vi "testConnectDisconnect.vi"(8 "error in (no error)":errorcluster) -> (0 "error out":errorcluster)   [LabVIEW 2018]
doc: "This VI test the connection and disconnection of TcpServerCmd and TcpServerTel."
uses:
  <vilib>/addons/_JKI Toolkits/Caraya/classes/Assert/Assert Equal Value_Variant.vi
  src/TcpServer/TcpServer.lvclass
  <vilib>/addons/_JKI Toolkits/Caraya/classes/Test/Test.lvclass
  <vilib>/addons/_JKI Toolkits/Caraya/classes/Assert/Assert.lvclass
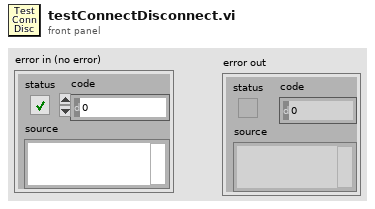
[diagram p1: front panel]
types:
  T1 = cluster{"CmdRead":refnum<user-event>, "EvtRead":refnum<user-event>, "GenRead":refnum<user-event>}
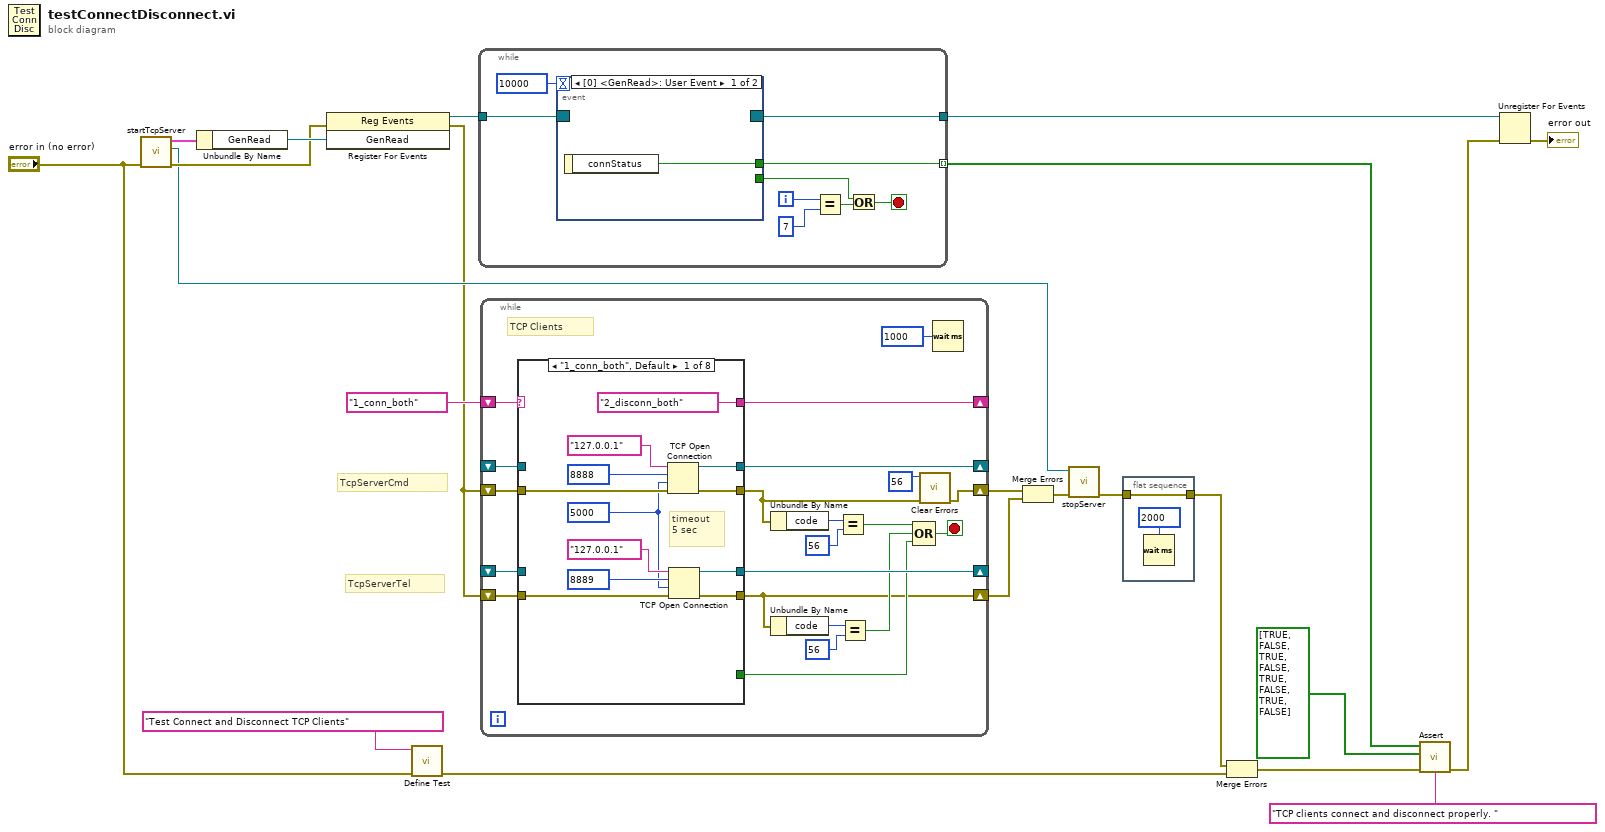
[diagram p0: block diagram]
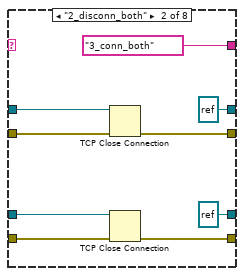
[diagram p2: hidden frame]
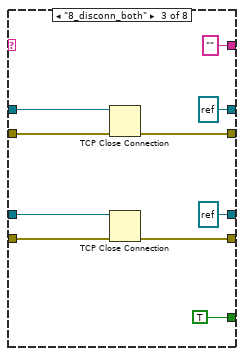
[diagram p3: hidden frame]
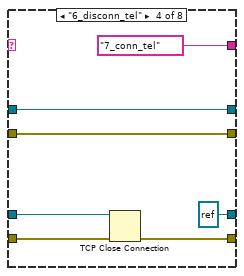
[diagram p4: hidden frame]
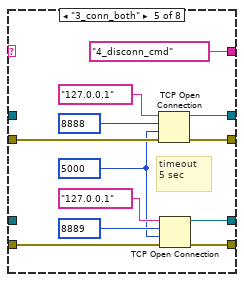
[diagram p5: hidden frame]
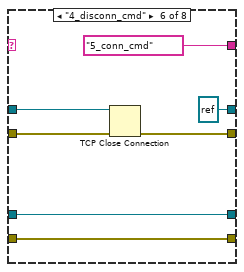
[diagram p6: hidden frame]
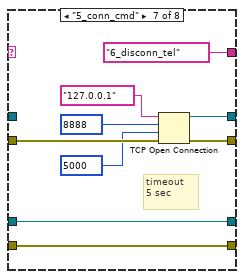
[diagram p7: hidden frame]
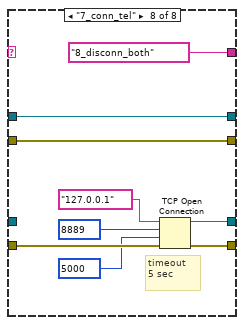
[diagram p8: hidden frame]
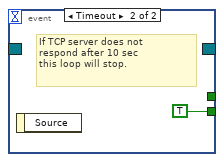
[diagram p9: hidden frame]
diagram:
  # "TcpServerTel"
  # "TcpServerCmd"
  n1 = call "startTcpServer.vi"("error in (no error)"="error in (no error)") -> ("error out"=w14:errorcluster, "TcpServer out"=w10:refnum<class "TcpServer.lvclass">, "UserEvents"=w17:T1)  [unwired: 8 in]
  n2 = Unbundle By Name(w17) -> ("GenRead"=w16:refnum<user-event>)
  n3 = register-events(error in=w14, w16) -> (reference out=w22:refnum<event-registration>, error out=w2:errorcluster)  [unwired: 1 in]
  n4 = call <vilib>:"Define Test.vi"("error in (no error)"="error in (no error)", "Label (VI Title)"="Test Connect and Disconnect TCP Clients") -> ("error out"=w7:errorcluster)  [unwired: 9 in]
  n5 = while {
    tunnel: w22 -> [w31]
    tunnel: [w30] -> w21
    tunnel: [w27] -> w9 mode=indexing
    i -> [w28]
    stop <- w23 stop-if-true
    n6 = event shown="[0] <GenRead>: User Event" {
      selector: w31 -> [_ _]
      dyn-events: [_ _] -> w30
      timeout: 10000 -> [_ _]
      tunnel: [w32 _] -> w27
      tunnel: [_ TRUE] -> w24
      event User Event {
        n7 = event-data() -> ("connStatus"=w32:bool)  [unwired: 1 in]
      }
      event Timeout {
        # "If TCP server does not\nrespond after 10 sec\nthis loop will stop."
        n8 = event-data() -> ()  [unwired: 1 in, 1 out]
      }
    }
    n9 = Equal?(x=w28, y=7) -> (x = y?=w25:bool)
    n10 = Or(x=w24, y=w25) -> (x .or. y?=w23:bool)
  }
  n11 = while {
    shift-right: [w47] -> _
    shift-left: "1_conn_both" ("address") -> [w54]
    shift-right: [w53] -> _
    shift-left: _ -> [w51]
    shift-right: [w52] -> _
    shift-left: _ -> [w50]
    shift-right: [w40] -> w13
    shift-left: w2 -> [w49]
    shift-right: [w35] -> w12
    shift-left: w2 -> [w48]
    stop <- w41 stop-if-true
    # "TCP Clients"
    n12 = case shown="\"1_conn_both\", Default" w54 {
      tunnel: [w62 refnum<k5> refnum ("connection ID") refnum<k5> refnum ("connection ID") w86 w100 refnum<k5> refnum ("connection ID") w118 w122] -> w53
      tunnel: [w61 refnum<k5> refnum ("connection ID") refnum<k5> refnum ("connection ID") refnum<k5> refnum ("connection ID") w99 w105 w113 w127] -> w52
      tunnel: w51 -> [_ w75 w85 w86 _ w111 _ w122]
      tunnel: w50 -> [_ w73 w83 w91 _ w105 w113 _]
      tunnel: [w60 w71 w81 w92 w98 w108 w117 w124] -> w37
      tunnel: [w59 w70 w80 w89 w97 w109 w114 w126] -> w35
      tunnel: w49 -> [w57 w74 w84 w92 w95 w110 w115 w124]
      tunnel: w48 -> [w56 w72 w82 w90 w94 w109 w114 w123]
      tunnel: ["2_disconn_both" ("address") "3_conn_both" ("address") "" ("address") "7_conn_tel" ("address") "4_disconn_cmd" ("address") "5_conn_cmd" ("address") "6_disconn_tel" ("address") "8_disconn_both" ("address")] -> w47
      tunnel: [_ _ TRUE _ _ _ _ _] -> w38
      frame "1_conn_both", Default {
        w55 = 5000 ("timeout ms (60000)")
        # "timeout\n5 sec"
        n13 = TCP Open Connection(address="127.0.0.1", remote port or service name=u16 8888, timeout ms (60000)=w55, error in (no error)=w57) -> (connection ID=w62:refnum<k5>, error out=w60:errorcluster)  [unwired: 1 in]
        n14 = TCP Open Connection(address="127.0.0.1", remote port or service name=u16 8889, timeout ms (60000)=w55, error in (no error)=w56) -> (connection ID=w61:refnum<k5>, error out=w59:errorcluster)  [unwired: 1 in]
      }
      frame "2_disconn_both" {
        n15 = TCP Close Connection(connection ID=w75, error in (no error)=w74) -> (error out=w71:errorcluster)  [unwired: 1 in, 1 out]
        n16 = TCP Close Connection(connection ID=w73, error in (no error)=w72) -> (error out=w70:errorcluster)  [unwired: 1 in, 1 out]
      }
      frame "8_disconn_both" {
        n17 = TCP Close Connection(connection ID=w85, error in (no error)=w84) -> (error out=w81:errorcluster)  [unwired: 1 in, 1 out]
        n18 = TCP Close Connection(connection ID=w83, error in (no error)=w82) -> (error out=w80:errorcluster)  [unwired: 1 in, 1 out]
      }
      frame "6_disconn_tel" {
        n19 = TCP Close Connection(connection ID=w91, error in (no error)=w90) -> (error out=w89:errorcluster)  [unwired: 1 in, 1 out]
      }
      frame "3_conn_both" {
        w93 = 5000 ("timeout ms (60000)")
        # "timeout\n5 sec"
        n20 = TCP Open Connection(address="127.0.0.1", remote port or service name=u16 8888, timeout ms (60000)=w93, error in (no error)=w95) -> (connection ID=w100:refnum<k5>, error out=w98:errorcluster)  [unwired: 1 in]
        n21 = TCP Open Connection(address="127.0.0.1", remote port or service name=u16 8889, timeout ms (60000)=w93, error in (no error)=w94) -> (connection ID=w99:refnum<k5>, error out=w97:errorcluster)  [unwired: 1 in]
      }
      frame "4_disconn_cmd" {
        n22 = TCP Close Connection(connection ID=w111, error in (no error)=w110) -> (error out=w108:errorcluster)  [unwired: 1 in, 1 out]
      }
      frame "5_conn_cmd" {
        # "timeout\n5 sec"
        n23 = TCP Open Connection(address="127.0.0.1", remote port or service name=u16 8888, timeout ms (60000)=5000, error in (no error)=w115) -> (connection ID=w118:refnum<k5>, error out=w117:errorcluster)  [unwired: 1 in]
      }
      frame "7_conn_tel" {
        # "timeout\n5 sec"
        n24 = TCP Open Connection(address="127.0.0.1", remote port or service name=u16 8889, timeout ms (60000)=5000, error in (no error)=w123) -> (connection ID=w127:refnum<k5>, error out=w126:errorcluster)  [unwired: 1 in]
      }
    }
    n25 = Unbundle By Name(w37) -> ("code"=w36:i32)
    n26 = Unbundle By Name(w35) -> ("code"=w34:i32)
    n27 = Equal?(x=w36, y=56) -> (x = y?=w43:bool)
    n28 = Equal?(x=w34, y=56) -> (x = y?=w42:bool)
    n29 = Compound Arithmetic op=OR(w43, w42, w38) -> (w41:bool)
    n30 = call <vilib>:"Clear Errors.vi"("error in (no error)"=w37, "specific error code to clear (0: all)"=56) -> ("error out"=w40:errorcluster)  [unwired: 4 in, 1 out]
    n31 = Wait (ms)(milliseconds to wait=u32 1000) -> ()  [unwired: 1 out]
  }
  n32 = Merge Errors(w13, w12) -> (w11:errorcluster)
  n33 = call "stopServer.vi"("error in (no error)"=w11, "tcpServer in"=w10) -> ("error out"=w19:errorcluster)  [unwired: 8 in, 1 out]
  n34 = flat-sequence {
    tunnel: w19 -> [w130]
    tunnel: [w130] -> w4
    frame #0 {
      n35 = Wait (ms)(milliseconds to wait=u32 2000) -> ()  [unwired: 1 out]
    }
  }
  n36 = Merge Errors(w4, w7) -> (w5:errorcluster)
  n37 = call-poly <vilib>:"Assert.vi"("Label"="TCP clients connect and disconnect properly. ", "error in (no error)"=w5, "Y"=bool[] [TRUE, FALSE, TRUE, FALSE, TRUE, FALSE, TRUE, FALSE], "X"=w9) -> ("error out"=w6:errorcluster)  [unwired: 7 in]
  n38 = Unregister For Events(event registration refnum=w21, error in=w6) -> (error out=→"error out":errorcluster)
